vi "DataLog Build Tag Entry Histogram.vi"(7 "aggregation entries in":T1[](array[typedef]) {"point"."value" format="%.3e"; "point"."time" format="%<%H:%M:%S%2u\n%Y/%m/%d>T"}, 11 "error in (no error)":errorcluster) -> (4 "entries per tag":i32[](array[numeric]), 8 "aggregation entries out":T1[](array[typedef]) {"point"."value" format="%.3e"; "point"."time" format="%<%H:%M:%S%2u\n%Y/%m/%d>T"}, 15 "dup error":errorcluster)   [LabVIEW 2012]
doc: "Counts the number of aggregation entries per tag. This allows recovery operations to be limited to those tags with entries in the aggregation buffer and recovery arrays to be preallocated with a sufficient but not excessive size."
uses:
  typedefs/clusters/t_DataLog Aggregation Entry.ctl
  typedefs/clusters/t_DataLog Point.ctl
  typedefs/t_DataLog Tag Hash Methods.ctl
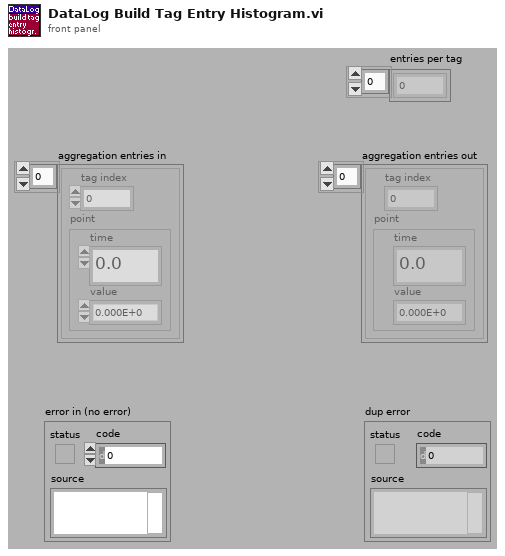
[diagram p1: front panel]
types:
  T1 = typedef "t_DataLog Aggregation Entry.ctl" = cluster{"tag index":i32, "point":T2}
  T2 = typedef "t_DataLog Point.ctl" = cluster{"time":dbl, "value":dbl}
  T3 = typedef "t_DataLog Tag Hash Methods.ctl" = enum16{"initialize", "add tag", "index tag", "lookup", "#tags", "cleanup", "write recovery", "read recovery", "delete recovery"}
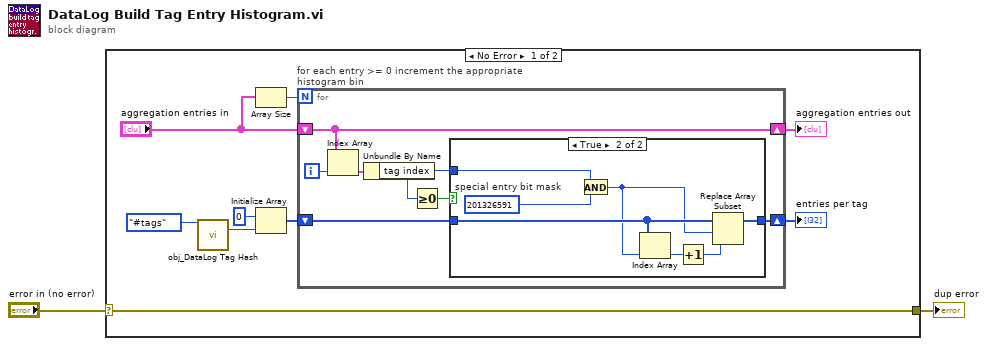
[diagram p0: block diagram]
diagram:
  n1 = case shown="No Error" "error in (no error)" {
    selector: "error in (no error)" -> [w11 w27]
    tunnel: [w11 w27] -> w2
    frame No Error {
      n2 = call "obj_DataLog Tag Hash.vi"("method"=t_DataLog_Tag_Hash_Methods."#tags") -> ("#tags"=w4:i32)  [unwired: 11 in, 3 out]
      n3 = Array Size(array="aggregation entries in") -> (size(s)=w10:i32)
      n4 = Initialize Array(0, w4) -> (w5:i32[])
      n5 = for "for each entry >= 0 increment the appropriate histogram bin" {
        N: w10 -> [_]
        shift-right: [w17] -> w7
        shift-left: "aggregation entries in" -> [w17]
        shift-right: [w12] -> w8
        shift-left: w5 -> [w13]
        i -> [w18]
        n6 = Index Array(array=w17, index=w18) -> (element=w16:T1)
        n7 = Unbundle By Name(w16) -> ("tag index"=w15:i32)
        n8 = Greater Or Equal To 0?(x=w15) -> (x >= 0?=w14:bool)
        n9 = case shown="True" w14 {
          tunnel: w15 -> [_ w21]
          tunnel: w13 -> [w19 w26]
          tunnel: [w19 w25] -> w12
          frame False {
          }
          frame True {
            w22 = 201326591  # special entry bit mask
            n10 = And(x=w21, y=w22) -> (x .and. y?=w20:i32)
            n11 = Index Array(array=w26, index=w20) -> (element=w24:i32)
            n12 = Increment(x=w24) -> (x+1=w23:i32)
            n13 = Replace Array Subset(array=w26, new element=w23, index=w20) -> (w25:i32[])
          }
        }
      }
      "aggregation entries out" <- w7
      "entries per tag" <- w8
    }
    frame Error {
    }
  }
  "dup error" <- w2
